vi "YSCS_CB.vi"(1 "校验码":u8 format="%02x", 3 "校验起始位":u32, 4 "输入字符串":string) -> (0 "输出字符串":string)   [LabVIEW 2015]
doc: "在任意的位置输出固定字节"
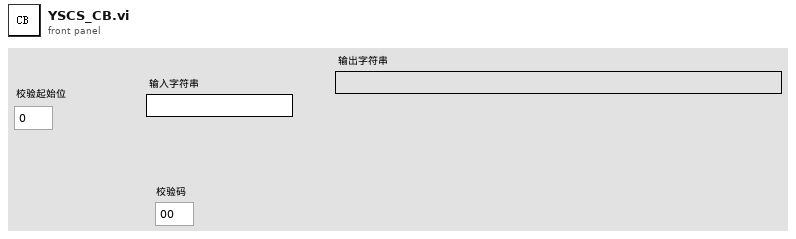
[diagram p1: front panel]
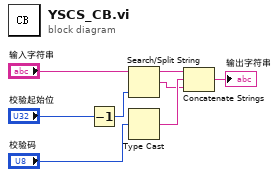
[diagram p0: block diagram]
diagram:
  n1 = Decrement(x="校验起始位") -> (x-1=w6:u32)
  n2 = Search/Split String(string="输入字符串", offset (0)=w6) -> (substring before match=w7:string, match + rest of string=w2:string)  [unwired: 1 in, 1 out]
  n3 = Type Cast(x="校验码") -> (*(type *) &x=w3:string)  [unwired: 1 in]
  n4 = Concatenate Strings(w7, w3, w2) -> (→"输出字符串":string)
